vi "Command (read & write) - RL.vi"(7 "timeout ms (100)":i32=100, 8 "error in (no error)":errorcluster, 9 "Register":string, 10 "IP":string, 11 "connection ID in":refnum<k16>) -> (0 "error out":errorcluster, 2 "Register Value":string, 3 "connection ID out":refnum<k16>)   [LabVIEW 2016, in "SMD-7615.lvlib" / "eSCL.lvlib"]
doc: "RL - Register Load - immediate\nSets or reads a data register to the given immediate data value. The data value is checked and stored as a Long word. When setting a Short-word register with the given Long-word data value only the lower word of the Long value is used.\nParameter\nR: Reads Register R\nR=100 : Sets Register R to 100\nBoth cases return the current (or newly set) register values"
uses:
  eSCL.lvlib
  String Command and Param.ctl
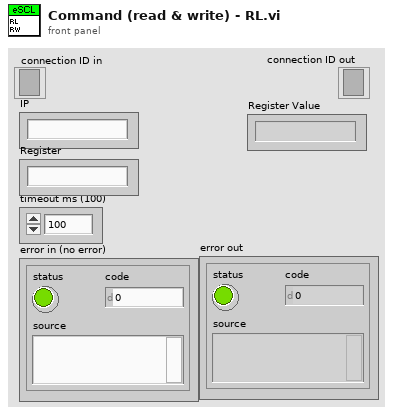
[diagram p1: front panel]
types:
  T1 = typedef "SMD-7615.lvlib/eSCL.lvlib/String Command and Param.ctl" = cluster{"Command":string, "String Parameler":string, "String Parameler Default":string}
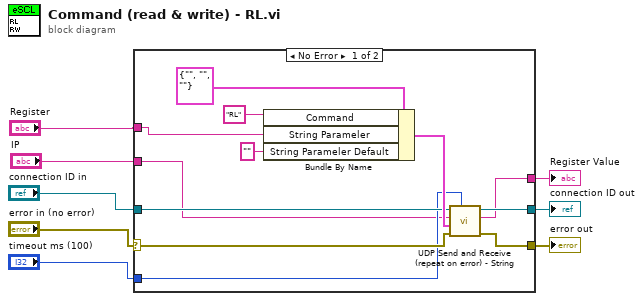
[diagram p0: block diagram]
diagram:
  n1 = case shown="No Error" "error in (no error)" {
    selector: "error in (no error)" -> [w15 w21]
    tunnel: "connection ID in" -> [w13 w22]
    tunnel: [w18 w22] -> w2
    tunnel: [w16 w21] -> w1
    tunnel: "IP" -> [w11 _]
    tunnel: "timeout ms (100)" -> [w12 _]
    tunnel: [w17 _] -> w3
    tunnel: "Register" -> [w10 _]
    frame No Error {
      n2 = Bundle By Name(cluster=T1 {"Command"="", "String Parameler"="", "String Parameler Default"=""} ("String Command & Param"), "Command"="RL", "String Parameler"=w10, "String Parameler Default"="") -> (w14:T1)
      n3 = call "UDP Send and Receive (repeat on error) - String.vi"("timeout ms (100)"=w12, "error in (no error)"=w15, "String Command & Param"=w14, "IP"=w11, "connection ID in"=w13) -> ("error out"=w16:errorcluster, "String Param out"=w17:string, "connection ID out"=w18:refnum<k16>)  [unwired: 4 in]
    }
    frame Error {
    }
  }
  "connection ID out" <- w2
  "error out" <- w1
  "Register Value" <- w3
